vi "Draw.vi"(8 "Error In":errorcluster, 9 "Coordinants":cluster{"X":i16, "Y":i16}, 10 "2D Picture In":picture, 11 "Circle in":refnum<class "Circle.lvclass">) -> (0 "Error Out":errorcluster, 2 "2D Picture Out":picture, 3 "Circle out":refnum<class "Circle.lvclass">)   [LabVIEW 2021, in "Circle.lvclass"]
doc: "Draw a circle on 2D picture.\nCoordinants is postion of circle center."
uses:
  Circle.lvclass
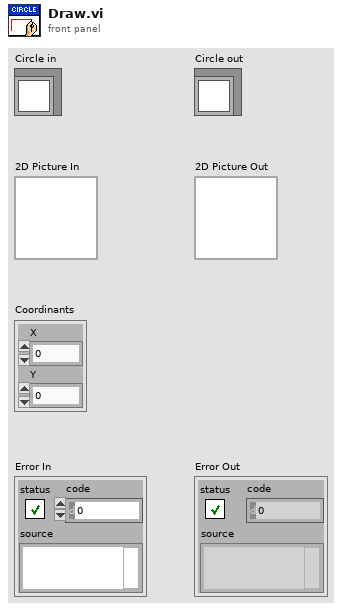
[diagram p1: front panel]
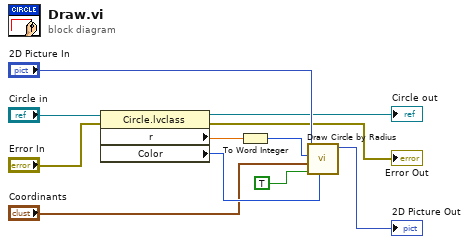
[diagram p0: block diagram]
diagram:
  n1 = property class="Circle.lvclass"(reference="Circle in", error in="Error In") -> (reference out=→"Circle out":refnum<class "Circle.lvclass">, error out=→"Error Out":errorcluster, "r"=w9:dbl, "Color"=w6:u32)
  n2 = To Word Integer(number=w9) -> (16bit integer=w8:i16)
  n3 = call <vilib>:"Draw Circle by Radius.vi"("color(black)"=w6, "fill?(F)"=TRUE, "pixel center"="Coordinants", "radius"=w8, "picture"="2D Picture In") -> ("new picture"=→"2D Picture Out":picture)  [unwired: 6 in]
